vi "main 4th.vi"() -> ()   [LabVIEW 2015]
uses:
  <vilib>/Utility/file.llb/Read From Spreadsheet File (DBL).vi
panel:
  out "数值 2":i32
  out "From OD fit?":bool
  out "Current file num":i32
  in  "Image Dark":dbl[][](array[numeric])
  in  "Image Light":dbl[][](array[numeric])
  in  "Image Atom":dbl[][](array[numeric])
  out "Best fit parameters":dbl[](array[numeric])
  out "Fitting Results Save Path":string[](array[string])
  out "Best fit results":dbl[][](array[numeric])
  in  "Initial guess values":dbl[](array[numeric])
  in  "Latest image data":dbl[][](array[numeric])
  out "Fitting Type":u16(ring)
  out "Force Guess?":bool
  out "Aquired?":bool
  out "ROI Height":u32
  out "ROI Width":u32
  out "OD image":dbl[][](graph)
  out "Process Index":i32
  out "External Trigger":bool
  out "XY图":cluster{i32[], dbl[]}[](graph)
  in  "OD fit":bool
  in  "OD num":i32
  out "Fit Done":bool
  in  "Exit":bool
  out "XY图 2":cluster{i32[], dbl[]}[](graph)
  in  "Auto Split":bool
  in  "Fit":bool
  in  "Open File":bool
  in  "Auto Fit":bool
  in  "Stop":bool
  in  "Aquire":bool
  in  "Fitting Config":bool
  in  "Camera Config":bool
  in  "Initialize":bool
  in  "Live Image Display":refnum<k7>(container)
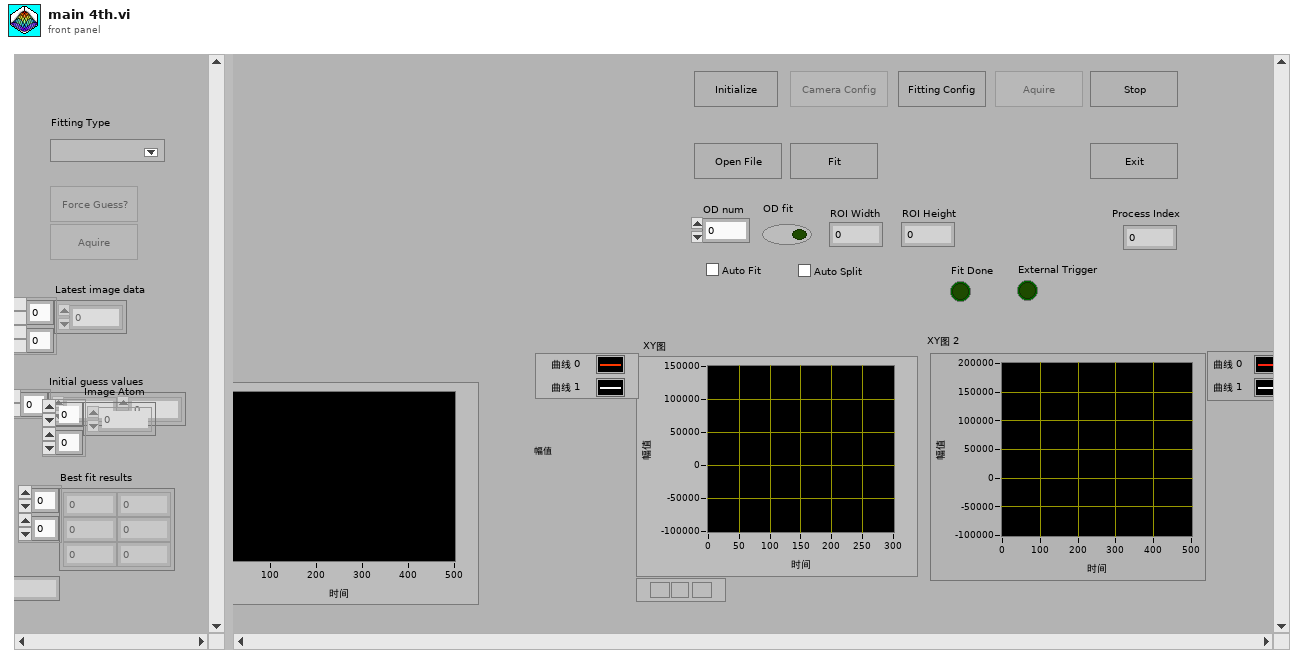
[diagram p1: front panel]
types:
  T1 = enum8{"Enabled", "Disabled", "Disabled and Grayed Out"}
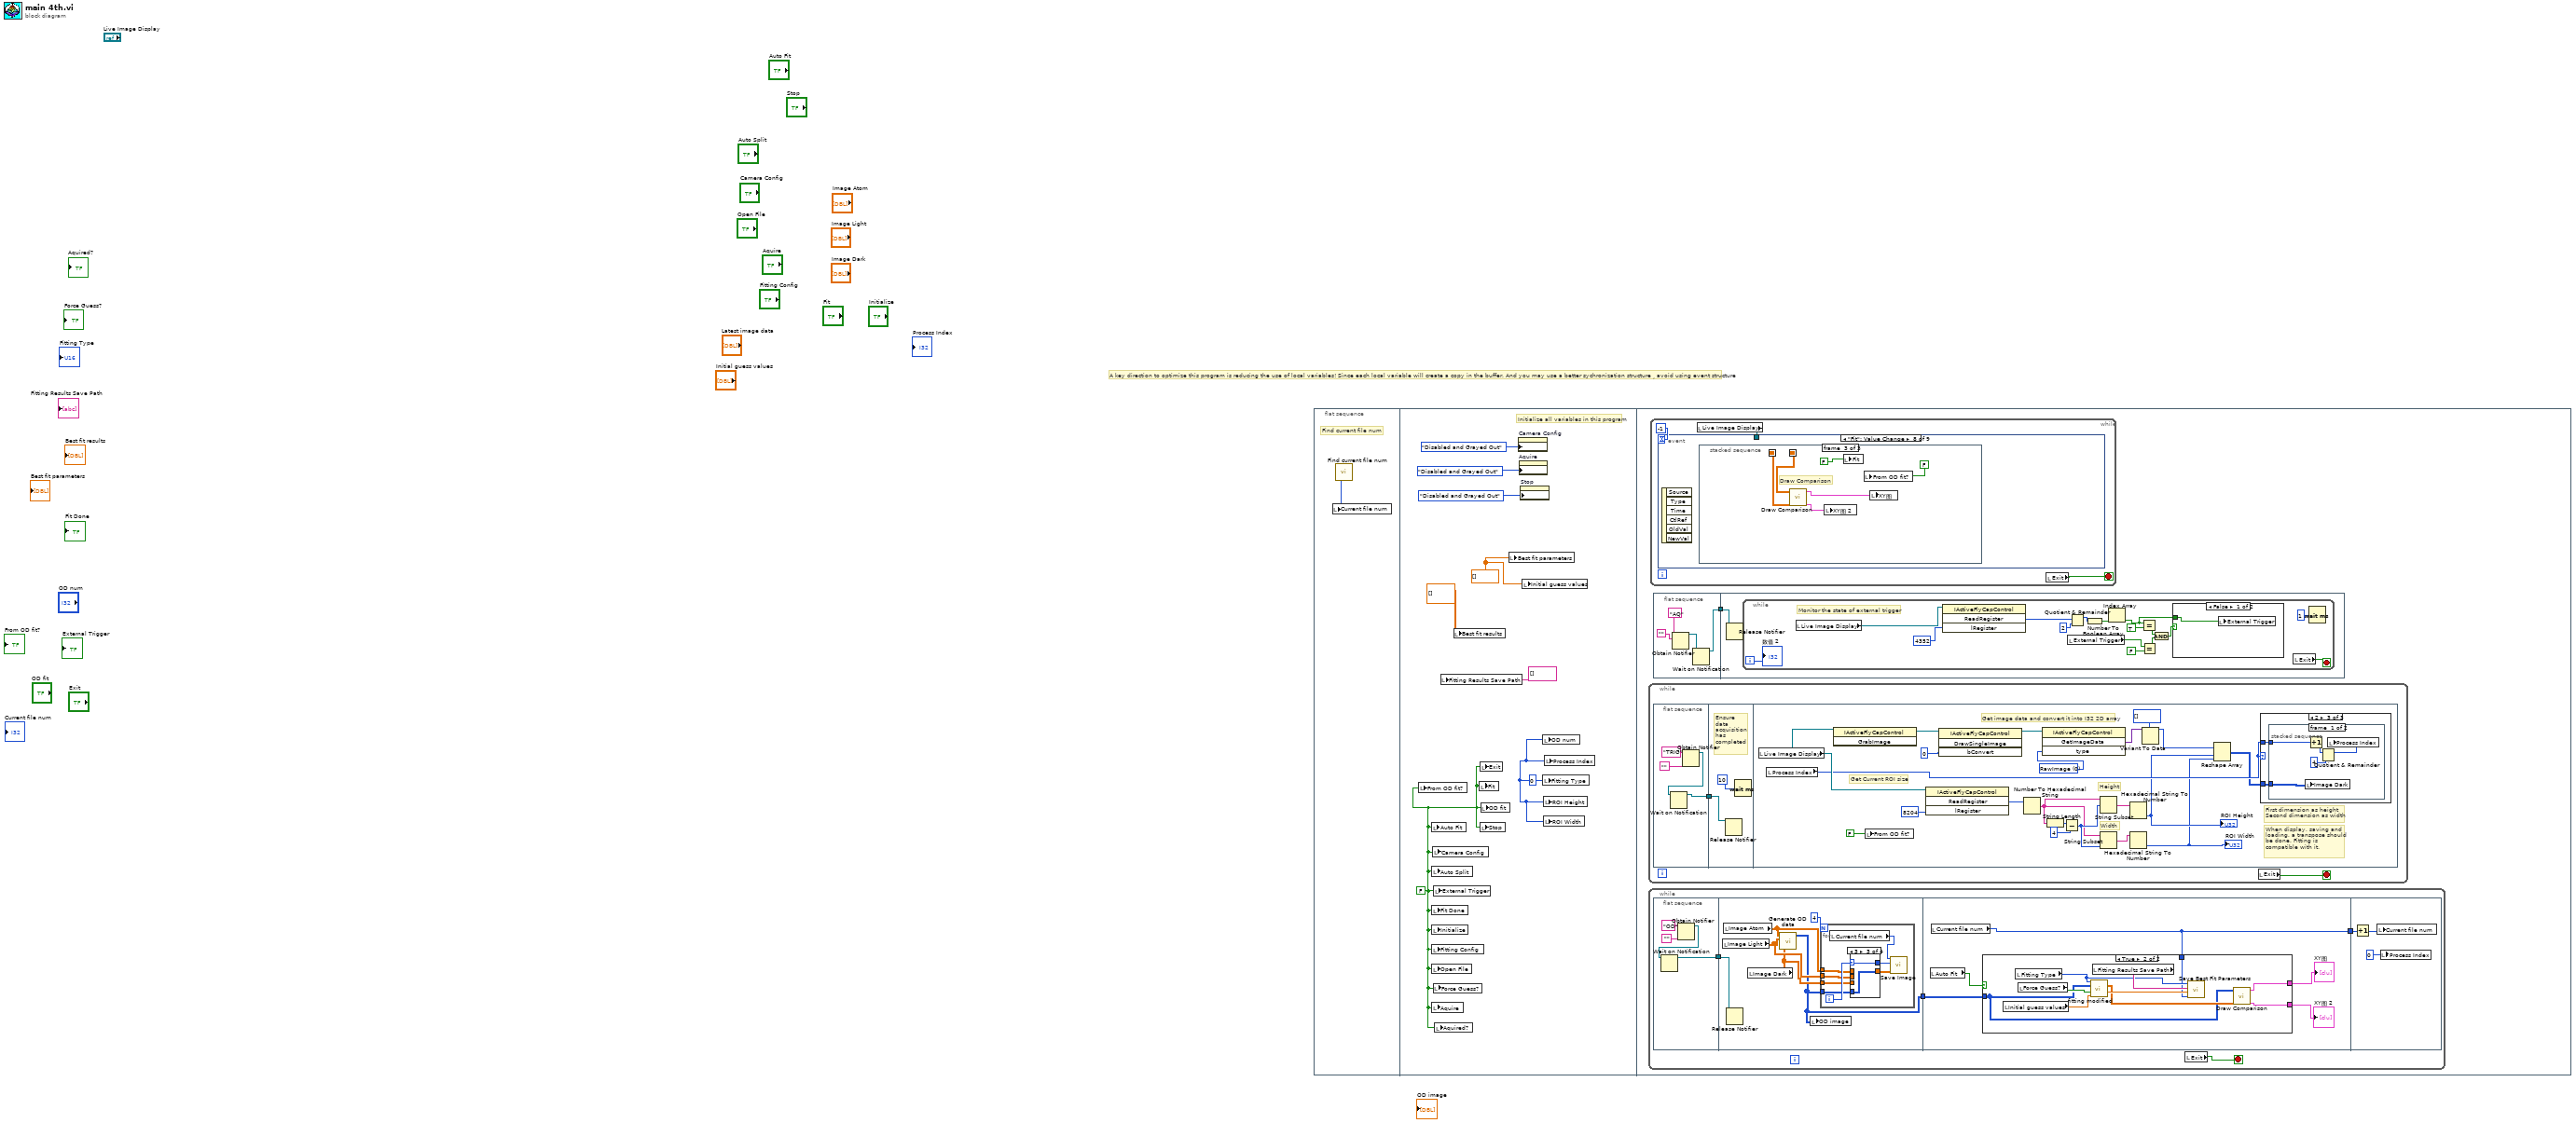
[diagram p0: block diagram]
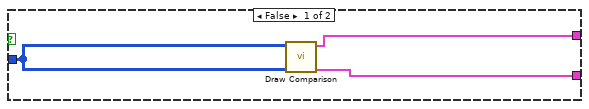
[diagram p5: hidden frame]
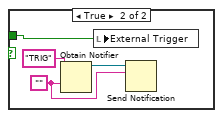
[diagram p6: hidden frame]
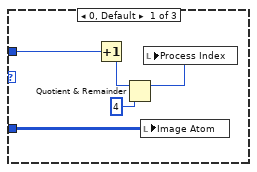
[diagram p7: hidden frame]
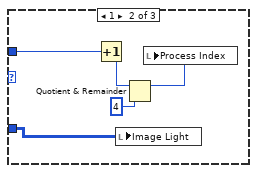
[diagram p8: hidden frame]
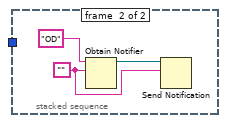
[diagram p9: hidden frame]
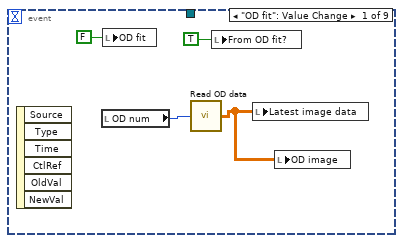
[diagram p10: hidden frame]
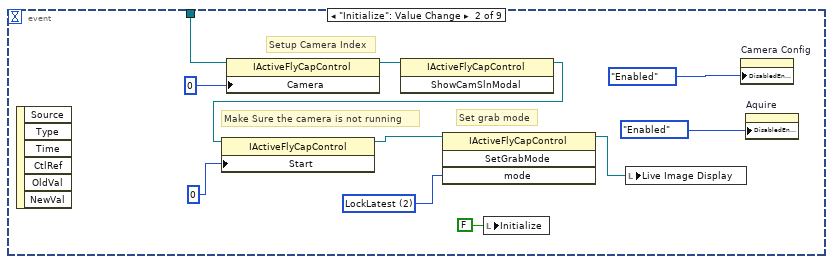
[diagram p11: hidden frame]
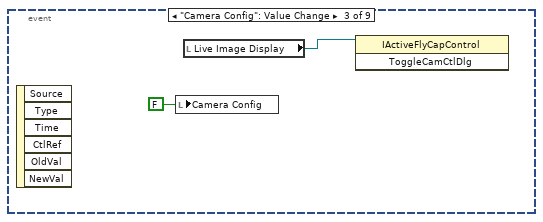
[diagram p12: hidden frame]
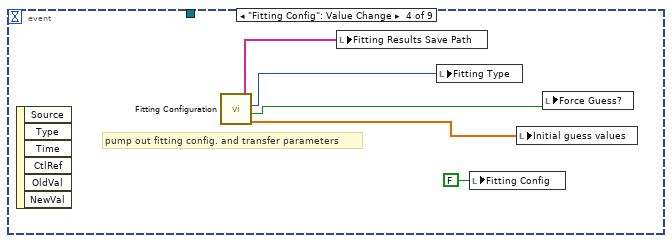
[diagram p13: hidden frame]
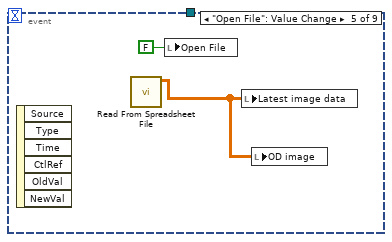
[diagram p14: hidden frame]
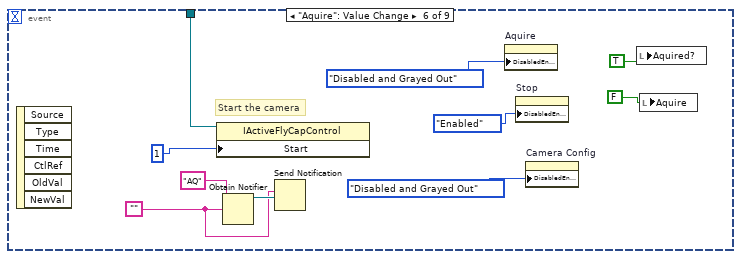
[diagram p15: hidden frame]
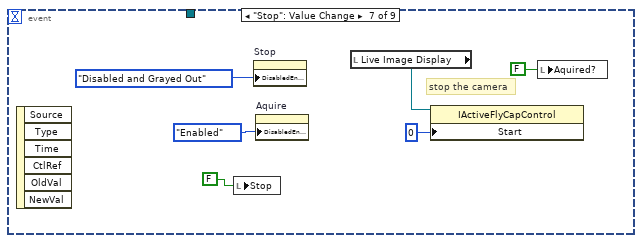
[diagram p16: hidden frame]
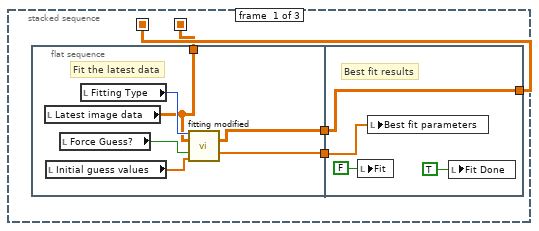
[diagram p17: hidden frame]
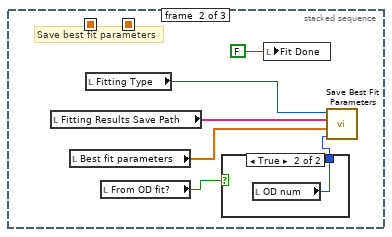
[diagram p18: hidden frame]
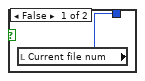
[diagram p19: hidden frame]
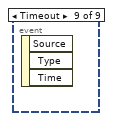
[diagram p20: hidden frame]
diagram:
  # "A key direction to optimize this program is reducing the use of local variables! Since each local variable will create a copy in the buffer. And you may use a better sychronization structure，avoid using event structure"
  n1 = flat-sequence {
    frame #0 {
      # "Find current file num"
      n2 = call "Find current file num.vi"() -> ("Current File Num"=w1:u16)  [unwired: 2 in]
      n3 = local write "Current file num"(w1) -> ()
    }
    frame #1 {
      w5 = 0 ("OD num")
      w4 = dbl[] [] ("Best fit parameters")
      w3 = FALSE ("Aquire")
      # "Initialize all variables in this program"
      n4 = local write "From OD fit?"(w3) -> ()
      n5 = local write "Auto Fit"(w3) -> ()
      n6 = local write "Auto Split"(w3) -> ()
      n7 = local write "Fit Done"(w3) -> ()
      n8 = local write "Initialize"(w3) -> ()
      n9 = local write "Fitting Config"(w3) -> ()
      n10 = local write "Open File"(w3) -> ()
      n11 = local write "Aquire"(w3) -> ()
      n12 = local write "Camera Config"(w3) -> ()
      n13 = local write "Force Guess?"(w3) -> ()
      n14 = local write "External Trigger"(w3) -> ()
      n15 = local write "Aquired?"(w3) -> ()
      n16 = local write "Fitting Results Save Path"(string[] [] ("Fitting Results Save Path")) -> ()
      n17 = local write "Best fit results"(dbl[][] [] ("Best fit results")) -> ()
      n18 = local write "Fit"(w3) -> ()
      n19 = local write "Exit"(w3) -> ()
      n20 = local write "Stop"(w3) -> ()
      n21 = local write "OD fit"(w3) -> ()
      n22 = local write "Best fit parameters"(w4) -> ()
      n23 = property on="Camera Config" class="Bool (strict)"("DisabledEnum"=T1."Disabled and Grayed Out" ("禁用")) -> ()  [unwired: 2 in, 2 out]
      n24 = property on="Aquire" class="Bool (strict)"("DisabledEnum"=T1."Disabled and Grayed Out" ("禁用")) -> ()  [unwired: 2 in, 2 out]
      n25 = property on="Stop" class="Bool (strict)"("DisabledEnum"=T1."Disabled and Grayed Out" ("禁用")) -> ()  [unwired: 2 in, 2 out]
      n26 = local write "Initial guess values"(w4) -> ()
      n27 = local write "OD num"(w5) -> ()
      n28 = local write "Fitting Type"(w5) -> ()
      n29 = local write "ROI Height"(w5) -> ()
      n30 = local write "ROI Width"(w5) -> ()
      n31 = local write "Process Index"(w5) -> ()
    }
    frame #2 {
      n32 = while {
        stop <- w89 stop-if-true
        n33 = flat-sequence {
          tunnel: [w90] -> w88
          tunnel: w88 -> [w95]
          frame #0 {
            n34 = Obtain Notifier(name (unnamed)="TRIG" ("名称（未命名）"), notification data type="") -> (notifier out=w91:refnum<notifier>)  [unwired: 2 in, 2 out]
            n35 = Wait on Notification(notifier=w91) -> (notifier out=w90:refnum<notifier>)  [unwired: 3 in, 3 out]
          }
          frame #1 {
            # "Ensure\ndata\nacquisition\nhas \ncompleted"
            n36 = Release Notifier(notifier=w95) -> ()  [unwired: 2 in, 3 out]
            n37 = Wait (ms)(milliseconds to wait=u32 10 ("等待时间（毫秒）")) -> ()  [unwired: 1 out]
          }
          frame #2 {
            w116 = 0 items=["RawImage", "ColorProcessedImage"] ("type")
            # "Get image data and convert it into I32 2D array"
            # "When display, saving and \nloading, a transpose should\nbe done. Fitting is \ncompatible with it."
            # "First dimension as height\nSecond dimension as width"
            # "Width"
            # "Height"
            # "Get Current ROI size"
            n38 = local read "Live Image Display"() -> (w103:refnum<k7>)
            n39 = local read "Process Index"() -> (w99:i32)
            n40 = invoke class="IActiveFlyCapControl" method="GrabImage"(reference=w103) -> (reference out=w101:refnum<k7>)  [unwired: 2 in, 2 out]
            n41 = local write "From OD fit?"(FALSE ("From OD fit?")) -> ()
            n42 = invoke class="IActiveFlyCapControl" method="ReadRegister"(reference=w103, "lRegister"=u32 8204) -> ("ReadRegister"=w113:u32)  [unwired: 2 in, 3 out]
            n43 = invoke class="IActiveFlyCapControl" method="DrawSingleImage"(reference=w101, "bConvert"=0) -> (reference out=w102:refnum<k7>)  [unwired: 2 in, 3 out]
            n44 = Number To Hexadecimal String(2:w113) -> (0:w109:string)  [unwired: 1 in]
            n45 = invoke class="IActiveFlyCapControl" method="GetImageData"(reference=w102, "type"=w116) -> ("GetImageData"=w114:variant)  [unwired: 2 in, 3 out]
            n46 = String Length(string=w109) -> (length=w112:i32)
            n47 = Subtract(x=w112, y=4) -> (x-y=w110:i32)
            n48 = String Subset(string=w109, length (rest)=w110) -> (substring=w106:string)  [unwired: 1 in]
            n49 = String Subset(string=w109, offset (0)=w110) -> (substring=w107:string)  [unwired: 1 in]
            n50 = Hexadecimal String To Number(string=w106) -> (number=w96:u32)  [unwired: 2 in, 1 out]
            "ROI Width" <- w96
            n51 = Hexadecimal String To Number(string=w107) -> (number=w97:u32)  [unwired: 2 in, 1 out]
            "ROI Height" <- w97
            n52 = Variant To Data(type=i32[] [], Variant=w114) -> (data=w105:i32[])  [unwired: 1 in, 1 out]
            n53 = Reshape Array(w105, w97, w96) -> (w98:i32[][])
            n54 = case shown="2" w99 {
              tunnel: w99 -> [w118 w123 w128]
              tunnel: w98 -> [w117 w122 w127]
              frame 0, Default {
                n55 = Increment(x=w118) -> (x+1=w119:i32)
                n56 = Quotient & Remainder(x=w119, y=4) -> (x-y*floor(x/y)=w121:i32)  [unwired: 1 out]
                n57 = local write "Image Atom"(w117) -> ()
                n58 = local write "Process Index"(w121) -> ()
              }
              frame 1 {
                n59 = Increment(x=w123) -> (x+1=w124:i32)
                n60 = local write "Image Light"(w122) -> ()
                n61 = Quotient & Remainder(x=w124, y=4) -> (x-y*floor(x/y)=w126:i32)  [unwired: 1 out]
                n62 = local write "Process Index"(w126) -> ()
              }
              frame 2 {
                n63 = stacked-sequence {
                  tunnel: w128 -> [w130 _]
                  tunnel: w127 -> [w129 _]
                  frame #0 {
                    n64 = local write "Image Dark"(w129) -> ()
                    n65 = Increment(x=w130) -> (x+1=w131:i32)
                    n66 = Quotient & Remainder(x=w131, y=4) -> (x-y*floor(x/y)=w133:i32)  [unwired: 1 out]
                    n67 = local write "Process Index"(w133) -> ()
                  }
                  frame #1 {
                    w134 = ""
                    n68 = Obtain Notifier(name (unnamed)="OD" ("名称（未命名）"), notification data type=w134) -> (notifier out=w136:refnum<notifier>)  [unwired: 2 in, 2 out]
                    n69 = Send Notification(notification=w134, notifier=w136) -> ()  [unwired: 1 in, 2 out]
                  }
                }
              }
            }
          }
        }
        n70 = local read "Exit"() -> (w89:bool)
      }
      n71 = while {
        stop <- w14 stop-if-true
        n72 = flat-sequence {
          tunnel: [w15] -> w13
          tunnel: w13 -> [w24]
          tunnel: [w19] -> w12
          tunnel: w12 -> [w44]
          tunnel: [w43] -> w11
          tunnel: w11 -> [w60]
          frame #0 {
            n73 = Obtain Notifier(name (unnamed)="OD" ("名称（未命名）"), notification data type="") -> (notifier out=w16:refnum<notifier>)  [unwired: 2 in, 2 out]
            n74 = Wait on Notification(notifier=w16) -> (notifier out=w15:refnum<notifier>)  [unwired: 3 in, 3 out]
          }
          frame #1 {
            n75 = local read "Image Light"() -> (w22:dbl[][])
            n76 = local read "Image Atom"() -> (w23:dbl[][])
            n77 = Release Notifier(notifier=w24) -> ()  [unwired: 2 in, 3 out]
            n78 = local read "Image Dark"() -> (w21:dbl[][])
            n79 = call "Generate OD data.vi"("dark"=w21, "light"=w22, "atom"=w23) -> ("OD image"=w19:u16[][])  [unwired: 3 in]
            n80 = local write "OD image"(w19) -> ()
            n81 = for {
              N: 4 -> [_]
              tunnel: w23 -> [w31]
              tunnel: w22 -> [w30]
              tunnel: w21 -> [w29]
              tunnel: w19 -> [w28]
              i -> [w32]
              n82 = local read "Current file num"() -> (w26:i32)
              n83 = case shown="3" w32 {
                selector: w32 -> [w34 w36 w38 w40]
                tunnel: w31 -> [w33 _ _ _]
                tunnel: w30 -> [_ _ _ w39]
                tunnel: w29 -> [_ w35 _ _]
                tunnel: w28 -> [_ _ w37 _]
                tunnel: [w34 w36 w38 w40] -> w27
                tunnel: [w33 w35 w37 w39] -> w25
                frame 0, Default {
                }
                frame 2 {
                }
                frame 3 {
                }
                frame 1 {
                }
              }
              n84 = call "Save Image.vi"("Data"=w25, "Process Index"=w27, "Current File Num"=w26) -> ()  [unwired: 9 in]
            }
          }
          frame #2 {
            n85 = local read "Auto Fit"() -> (w45:bool)
            n86 = local read "Current file num"() -> (w43:i32)
            n87 = case shown="True" w45 {
              tunnel: w44 -> [w48 w51]
              tunnel: w43 -> [_ w53]
              tunnel: [w47 w50] -> w42
              tunnel: [w46 w49] -> w41
              frame False {
                n88 = call "Draw Comparison.vi"("Best Fit"=w48, "Raw Data"=w48) -> ("Vertical Comparison"=w46:cluster{i32[], dbl[]}[], "Horizontal Comparison"=w47:cluster{i32[], dbl[]}[])  [unwired: 7 in]
              }
              frame True {
                n89 = local read "Initial guess values"() -> (w57:dbl[])
                n90 = local read "Fitting Type"() -> (w54:u16)
                n91 = local read "Force Guess?"() -> (w58:bool)
                n92 = call "fitting modified.vi"("fitting type"=w54, "2D data"=w51, "force guess?"=w58, "intial guess value"=w57) -> ("best fit"=w52:dbl[][], "best fit parameters"=w56:dbl[])  [unwired: 8 in, 2 out]
                n93 = local read "Fitting Results Save Path"() -> (w55:string[])
                n94 = call "Save Best Fit Parameters.vi"("Current File Num"=w53, "Best Fit Parameters"=w56, "Fitting Results Save Path"=w55, "Fitting Type"=w54) -> ()  [unwired: 8 in]
                n95 = call "Draw Comparison.vi"("Best Fit"=w52, "Raw Data"=w51) -> ("Vertical Comparison"=w49:cluster{i32[], dbl[]}[], "Horizontal Comparison"=w50:cluster{i32[], dbl[]}[])  [unwired: 7 in]
              }
            }
            "XY图" <- w42
            "XY图 2" <- w41
          }
          frame #3 {
            n96 = Increment(x=w60) -> (x+1=w61:i32)
            n97 = local write "Current file num"(w61) -> ()
            n98 = local write "Process Index"(0 ("Process Index")) -> ()
          }
        }
        n99 = local read "Exit"() -> (w14:bool)
      }
      n100 = while {
        stop <- w138 stop-if-true
        n101 = local read "Live Image Display"() -> (w139:refnum<k7>)
        n102 = event shown="[7] \"Fit\": Value Change" {
          selector: _ -> [_ _ _ _ _ _ _ _ _]
          dyn-events: _ -> [_ _ _ _ _ _ _ _ _]
          timeout: -1 -> [_ _ _ _ _ _ _ _ _]
          tunnel: w139 -> [_ w148 _ _ _ w164 _ _ _]
          event "OD fit": Value Change {
            n103 = event-data() -> ()  [unwired: 1 in, 6 out]
            n104 = local read "OD num"() -> (w142:i32)
            n105 = local write "OD fit"(FALSE ("OD fit")) -> ()
            n106 = call "Read OD data.vi"("OD num"=w142) -> ("OD data"=w140:dbl[][])  [unwired: 4 in]
            n107 = local write "From OD fit?"(TRUE ("From OD fit?")) -> ()
            n108 = local write "Latest image data"(w140) -> ()
            n109 = local write "OD image"(w140) -> ()
          }
          event "Initialize": Value Change {
            w152 = 2 items=["FreeRunning", "LockNext", "LockLatest"] ("mode")
            # "Setup Camera Index"
            # "Set grab mode"
            # "Make Sure the camera is not running"
            n110 = event-data() -> ()  [unwired: 1 in, 6 out]
            n111 = property class="IActiveFlyCapControl"(reference=w148, "Camera"=0 ("Start")) -> (reference out=w151:refnum<k7>)  [unwired: 1 in, 1 out]
            n112 = invoke class="IActiveFlyCapControl" method="ShowCamSlnModal"(reference=w151) -> (reference out=w147:refnum<k7>)  [unwired: 2 in, 2 out]
            n113 = property class="IActiveFlyCapControl"(reference=w147, "Start"=0 ("Camera")) -> (reference out=w146:refnum<k7>)  [unwired: 1 in, 1 out]
            n114 = invoke class="IActiveFlyCapControl" method="SetGrabMode"(reference=w146, "mode"=w152) -> (reference out=w144:refnum<k7>)  [unwired: 2 in, 3 out]
            n115 = local write "Initialize"(FALSE ("Initialize")) -> ()
            n116 = local write "Live Image Display"(w144) -> ()
            n117 = property on="Camera Config" class="Bool (strict)"("DisabledEnum"=T1."Enabled" ("禁用")) -> ()  [unwired: 2 in, 2 out]
            n118 = property on="Aquire" class="Bool (strict)"("DisabledEnum"=T1."Enabled" ("禁用")) -> ()  [unwired: 2 in, 2 out]
          }
          event "Camera Config": Value Change {
            n119 = event-data() -> ()  [unwired: 1 in, 6 out]
            n120 = local write "Camera Config"(FALSE ("Camera Config")) -> ()
            n121 = local read "Live Image Display"() -> (w155:refnum<k7>)
            n122 = invoke class="IActiveFlyCapControl" method="ToggleCamCtlDlg"(reference=w155) -> ()  [unwired: 2 in, 3 out]
          }
          event "Fitting Config": Value Change {
            # "pump out fitting config. and transfer parameters"
            n123 = event-data() -> ()  [unwired: 1 in, 6 out]
            n124 = call "Fitting Configuration.vi"() -> ("intial guess"=w157:dbl[], "Force Guess？"=w158:bool, "Fitting Type"=w160:u16, "Fitting Results Save Path"=w159:string[])  [unwired: 5 in]
            n125 = local write "Fitting Results Save Path"(w159) -> ()
            n126 = local write "Fitting Type"(w160) -> ()
            n127 = local write "Fitting Config"(FALSE ("Fitting Config")) -> ()
            n128 = local write "Initial guess values"(w157) -> ()
            n129 = local write "Force Guess?"(w158) -> ()
          }
          event "Open File": Value Change {
            n130 = event-data() -> ()  [unwired: 1 in, 6 out]
            n131 = call-poly <vilib>:"Read From Spreadsheet File.vi"() -> ("all rows"=w162:dbl[][])  [unwired: 7 in, 4 out]
            n132 = local write "Open File"(FALSE ("Open File")) -> ()
            n133 = local write "Latest image data"(w162) -> ()
            n134 = local write "OD image"(w162) -> ()
          }
          event "Aquire": Value Change {
            w166 = ""
            # "Start the camera"
            n135 = event-data() -> ()  [unwired: 1 in, 6 out]
            n136 = property class="IActiveFlyCapControl"(reference=w164, "Start"=1) -> ()  [unwired: 1 in, 2 out]
            n137 = Obtain Notifier(name (unnamed)="AQ" ("名称（未命名）"), notification data type=w166) -> (notifier out=w167:refnum<notifier>)  [unwired: 2 in, 2 out]
            n138 = Send Notification(notification=w166, notifier=w167) -> ()  [unwired: 1 in, 2 out]
            n139 = property on="Aquire" class="Bool (strict)"("DisabledEnum"=T1."Disabled and Grayed Out" ("禁用")) -> ()  [unwired: 2 in, 2 out]
            n140 = property on="Stop" class="Bool (strict)"("DisabledEnum"=T1."Enabled" ("禁用")) -> ()  [unwired: 2 in, 2 out]
            n141 = property on="Camera Config" class="Bool (strict)"("DisabledEnum"=T1."Disabled and Grayed Out" ("禁用")) -> ()  [unwired: 2 in, 2 out]
            n142 = local write "Aquired?"(TRUE ("Aquired?")) -> ()
            n143 = local write "Aquire"(FALSE ("Initialize")) -> ()
          }
          event "Stop": Value Change {
            # "stop the camera"
            n144 = event-data() -> ()  [unwired: 1 in, 6 out]
            n145 = local write "Stop"(FALSE ("Initialize")) -> ()
            n146 = property on="Stop" class="Bool (strict)"("DisabledEnum"=T1."Disabled and Grayed Out" ("禁用")) -> ()  [unwired: 2 in, 2 out]
            n147 = property on="Aquire" class="Bool (strict)"("DisabledEnum"=T1."Enabled" ("禁用")) -> ()  [unwired: 2 in, 2 out]
            n148 = local read "Live Image Display"() -> (w175:refnum<k7>)
            n149 = property class="IActiveFlyCapControl"(reference=w175, "Start"=0) -> ()  [unwired: 1 in, 2 out]
            n150 = local write "Aquired?"(FALSE ("Aquired?")) -> ()
          }
          event "Fit": Value Change {
            n151 = event-data() -> ()  [unwired: 1 in, 6 out]
            n152 = stacked-sequence {
              seq-local: [w181 _ _] -> [_ _ w204]
              seq-local: [w180 _ _] -> [_ _ w202]
              frame #0 {
                n153 = flat-sequence {
                  tunnel: [w186] -> w183
                  tunnel: [w185] -> w182
                  tunnel: [w184] -> w180
                  tunnel: w183 -> [w190]
                  tunnel: w182 -> [w193]
                  tunnel: [w190] -> w181
                  frame #0 {
                    # "Fit the latest data"
                    n154 = local read "Latest image data"() -> (w184:dbl[][])
                    n155 = local read "Initial guess values"() -> (w188:dbl[])
                    n156 = local read "Force Guess?"() -> (w189:bool)
                    n157 = local read "Fitting Type"() -> (w187:u16)
                    n158 = call "fitting modified.vi"("fitting type"=w187, "2D data"=w184, "force guess?"=w189, "intial guess value"=w188) -> ("best fit"=w186:dbl[][], "best fit parameters"=w185:dbl[])  [unwired: 8 in, 2 out]
                  }
                  frame #1 {
                    # "Best fit results"
                    n159 = local write "Fit"(FALSE ("Fit")) -> ()
                    n160 = local write "Best fit parameters"(w193) -> ()
                    n161 = local write "Fit Done"(TRUE ("Fit Done")) -> ()
                  }
                }
              }
              frame #1 {
                # "Save best fit parameters"
                n162 = local read "Fitting Results Save Path"() -> (w197:string[])
                n163 = local read "Best fit parameters"() -> (w196:dbl[])
                n164 = local read "Fitting Type"() -> (w198:u16)
                n165 = local read "From OD fit?"() -> (w195:bool)
                n166 = case shown="True" w195 {
                  tunnel: [w200 w201] -> w194
                  frame False {
                    n167 = local read "Current file num"() -> (w200:i32)
                  }
                  frame True {
                    n168 = local read "OD num"() -> (w201:i32)
                  }
                }
                n169 = local write "Fit Done"(FALSE ("Fit Done")) -> ()
                n170 = call "Save Best Fit Parameters.vi"("Current File Num"=w194, "Best Fit Parameters"=w196, "Fitting Results Save Path"=w197, "Fitting Type"=w198) -> ()  [unwired: 8 in]
              }
              frame #2 {
                # "Draw Comparison"
                n171 = call "Draw Comparison.vi"("Best Fit"=w204, "Raw Data"=w202) -> ("Vertical Comparison"=w206:cluster{i32[], dbl[]}[], "Horizontal Comparison"=w207:cluster{i32[], dbl[]}[])  [unwired: 7 in]
                n172 = local write "XY图 2"(w206) -> ()
                n173 = local write "Fit"(FALSE ("Initialize")) -> ()
                n174 = local write "From OD fit?"(FALSE ("From OD fit?")) -> ()
                n175 = local write "XY图"(w207) -> ()
              }
            }
          }
          event Timeout {
            n176 = event-data() -> ()  [unwired: 1 in, 3 out]
          }
        }
        n177 = local read "Exit"() -> (w138:bool)
      }
      n178 = flat-sequence {
        tunnel: [w62] -> w10
        tunnel: w10 -> [w66]
        frame #0 {
          n179 = Obtain Notifier(name (unnamed)="AQ" ("名称（未命名）"), notification data type="") -> (notifier out=w64:refnum<notifier>)  [unwired: 2 in, 2 out]
          n180 = Wait on Notification(notifier=w64) -> (notifier out=w62:refnum<notifier>)  [unwired: 3 in, 3 out]
        }
        frame #1 {
          n181 = Release Notifier(notifier=w66) -> ()  [unwired: 2 in, 3 out]
          n182 = while {
            i -> [w81]
            stop <- w82 stop-if-true
            # "Monitor the state of external trigger"
            n183 = local read "Live Image Display"() -> (w80:refnum<k7>)
            n184 = invoke class="IActiveFlyCapControl" method="ReadRegister"(reference=w80, "lRegister"=u32 4352) -> ("ReadRegister"=w78:u32)  [unwired: 2 in, 3 out]
            n185 = local read "External Trigger"() -> (w73:bool)
            n186 = Quotient & Remainder(x=w78, y=u32 2) -> (x-y*floor(x/y)=w76:u32)  [unwired: 1 out]
            n187 = Number To Boolean Array(number=w76) -> (Boolean array=w75:bool[])
            n188 = Index Array(array=w75) -> (element=w68:bool)  [unwired: 1 in]
            n189 = Equal?(x=w68, y=TRUE) -> (x = y?=w70:bool)
            n190 = Equal?(x=w73, y=FALSE) -> (x = y?=w71:bool)
            n191 = And(x=w70, y=w71) -> (x .and. y?=w69:bool)
            n192 = case shown="False" w69 {
              tunnel: w68 -> [w83 w87]
              frame False {
                n193 = local write "External Trigger"(w83) -> ()
              }
              frame True {
                w84 = ""
                n194 = Obtain Notifier(name (unnamed)="TRIG" ("名称（未命名）"), notification data type=w84) -> (notifier out=w85:refnum<notifier>)  [unwired: 2 in, 2 out]
                n195 = local write "External Trigger"(w87) -> ()
                n196 = Send Notification(notification=w84, notifier=w85) -> ()  [unwired: 1 in, 2 out]
              }
            }
            n197 = local read "Exit"() -> (w82:bool)
            n198 = Wait (ms)(milliseconds to wait=u32 1 ("等待时间（毫秒）")) -> ()  [unwired: 1 out]
            "数值 2" <- w81
          }
        }
      }
    }
  }
